vi "Update Feedback.vi"(6 "Time":dbl, 8 "error in (no error)":errorcluster, 11 "2WayValve in":refnum<class "2WayValveH.lvclass">) -> (0 "error out":errorcluster, 3 "2WayValve out":refnum<class "2WayValveH.lvclass">)   [LabVIEW 2020, in "VolatusGUIElements.lvlib" / "2WayValveH.lvclass"]
uses:
  2WayValveH.lvclass
  2WayValveH.lvclass/2WayValveH.ctl
  lv-vecto/Vecto/Channel DBL/Channel DBL.lvclass/Channel DBL.ctl
  lv-vecto/Vecto/Group DBL/Value by Index.vi
  lv-vecto/Vecto/Channel DBL/Channel DBL.lvclass
  lv-vecto/Vecto/Vecto.lvlib
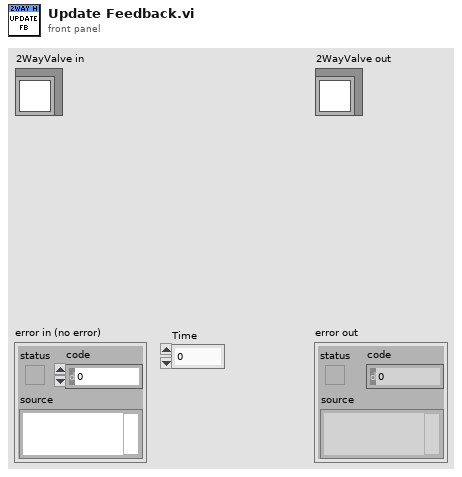
[diagram p1: front panel]
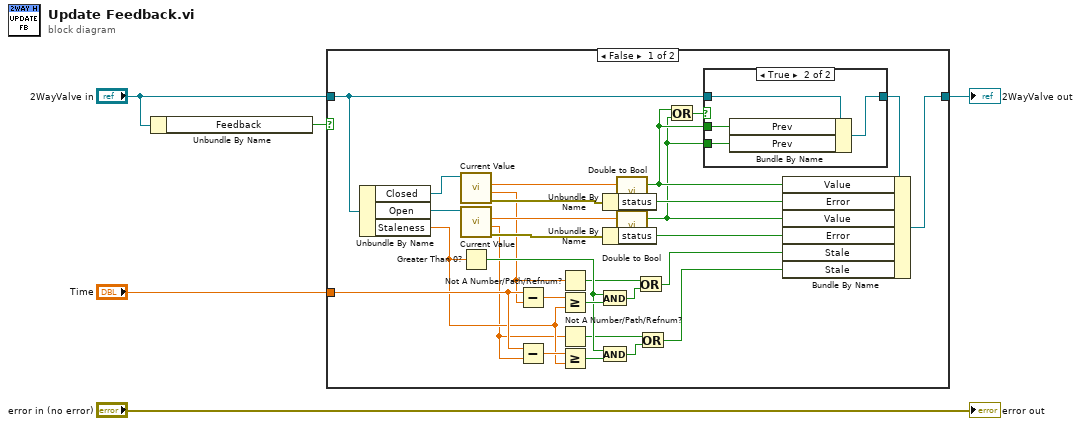
[diagram p0: block diagram]
diagram:
  n1 = Unbundle By Name("2WayValve in") -> ("Feedback"=w4:bool)
  n2 = case shown="False" w4 {
    tunnel: "2WayValve in" -> [w7 w40]
    tunnel: [w6 w40] -> w2
    tunnel: "Time" -> [w30 _]
    frame False {
      n3 = Unbundle By Name(w7) -> ("Closed"=w32:refnum<class "Channel DBL.lvclass">, "Open"=w31:refnum<class "Channel DBL.lvclass">, "Staleness"=w27:dbl)
      n4 = call "Current Value.vi"("Channel in"=w32) -> ("error out"=w34:errorcluster, "Timestamp"=w18:dbl, "Scaled"=w26:dbl)  [unwired: 6 in, 2 out]
      n5 = call "Current Value.vi"("Channel in"=w31) -> ("error out"=w33:errorcluster, "Timestamp"=w19:dbl, "Scaled"=w25:dbl)  [unwired: 6 in, 2 out]
      n6 = Greater Than 0?(x=w27) -> (x > 0?=w20:bool)
      n7 = Subtract(x=w30, y=w18) -> (x-y=w29:dbl)
      n8 = Subtract(x=w30, y=w19) -> (x-y=w28:dbl)
      n9 = Not A Number/Path/Refnum?(number/path/refnum=w18) -> (NaN/Path/Refnum?=w17:bool)
      n10 = Greater Or Equal?(x=w29, y=w27) -> (x >= y?=w22:bool)
      n11 = Not A Number/Path/Refnum?(number/path/refnum=w19) -> (NaN/Path/Refnum?=w14:bool)
      n12 = Greater Or Equal?(x=w28, y=w27) -> (x >= y?=w21:bool)
      n13 = And(x=w20, y=w22) -> (x .and. y?=w16:bool)
      n14 = And(x=w20, y=w21) -> (x .and. y?=w13:bool)
      n15 = Unbundle By Name(w34) -> ("status"=w24:bool)
      n16 = Unbundle By Name(w33) -> ("status"=w23:bool)
      n17 = call "Double to Bool.vi"("Double"=w26) -> ("Bool"=w10:bool)  [unwired: 2 in]
      n18 = call "Double to Bool.vi"("Double"=w25) -> ("Bool"=w9:bool)  [unwired: 2 in]
      n19 = Or(x=w17, y=w16) -> (x .or. y?=w15:bool)
      n20 = Or(x=w14, y=w13) -> (x .or. y?=w12:bool)
      n21 = Or(x=w10, y=w9) -> (x .or. y?=w11:bool)
      n22 = case shown="True" w11 {
        tunnel: w10 -> [_ w38]
        tunnel: w9 -> [_ w37]
        tunnel: w7 -> [w35 w39]
        tunnel: [w35 w36] -> w8
        frame False {
        }
        frame True {
          n23 = Bundle By Name(cluster=w39, "Prev"=w38, "Prev"=w37) -> (w36:refnum<class "2WayValveH.lvclass">)
        }
      }
      n24 = Bundle By Name(cluster=w8, "Value"=w10, "Error"=w24, "Value"=w9, "Error"=w23, "Stale"=w15, "Stale"=w12) -> (w6:refnum<class "2WayValveH.lvclass">)
    }
    frame True {
      # "Feedback unused"
    }
  }
  "2WayValve out" <- w2
  "error out" <- "error in (no error)"
